vi "Compute Control Dotted Name.vi"(10 "top control":refnum<vi>, 11 "control":refnum<vi>) -> (3 "dotted name":string[](array[string]))   [LabVIEW 2020]
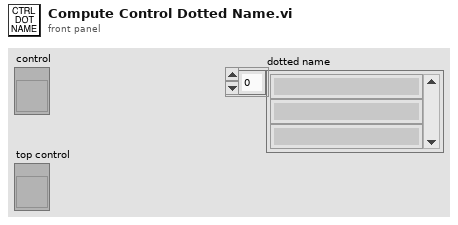
[diagram p1: front panel]
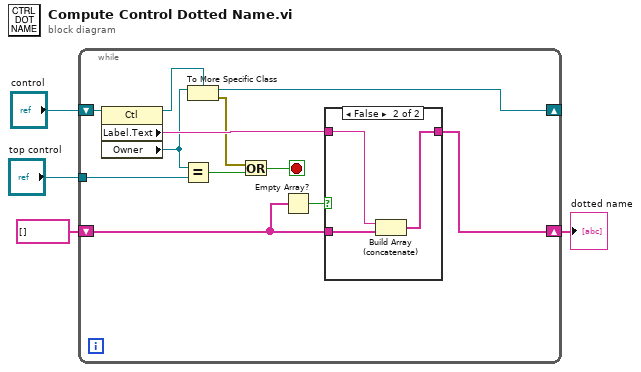
[diagram p0: block diagram]
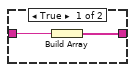
[diagram p2: hidden frame]
diagram:
  n1 = while {
    shift-right: [w15] -> w2
    shift-left: string[] [] -> [w5]
    tunnel: "top control" -> [w13]
    shift-right: [w10] -> _
    shift-left: "control" -> [w16]
    stop <- w7 stop-if-true
    n2 = property class="Ctl"(reference=w16) -> (reference out=w11:refnum<vi>, "Label.Text"=w14:string, "Owner"=w12:refnum<vi>)  [unwired: 1 in, 1 out]
    n3 = Equal?(x=w12, y=w13) -> (x = y?=w8:bool)
    n4 = To More Specific Class(target class=w11, reference=w12) -> (specific class reference=w10:refnum<vi>, error out=w9:errorcluster)  [unwired: 1 in]
    n5 = Or(x=w9, y=w8) -> (x .or. y?=w7:bool)
    n6 = Empty Array?(array=w5) -> (empty?=w6:bool)
    n7 = case shown="False" w6 {
      tunnel: [w17 w19] -> w15
      tunnel: w14 -> [w18 w21]
      tunnel: w5 -> [_ w20]
      frame True {
        n8 = Build Array(w18) -> (w17:string[])
      }
      frame False {
        n9 = Build Array (concatenate)(w21, w20) -> (w19:string[])
      }
    }
  }
  "dotted name" <- w2
